vi "Winch Drive.vi"(7 "Description":string, 8 "Command Info In":T1, 10 "Winch Motor":dbl) -> (0 "Command Info Out":T1)   [LabVIEW 2017]
doc: "This template is useful for immediate subsystem actions that do not need deadband filtering\n\nBe sure to right-click and select New from Template and save with a new command name."
uses:
  <vilib>/Rock Robotics/WPI/Framework/Command Status Info.ctl
  <vilib>/Rock Robotics/WPI/Framework/Completion Status.ctl
  <vilib>/Rock Robotics/WPI/Framework/Completion Notifier.ctl
  Implementation/Lift Setpoints.ctl
  Implementation/Lift Operations.ctl
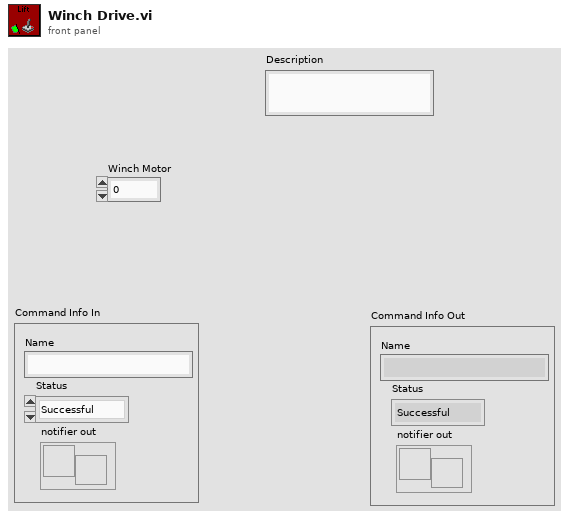
[diagram p1: front panel]
types:
  T1 = typedef "Command Status Info.ctl" = cluster{"Name":string, "Status":T2, "notifier out":T3}
  T2 = typedef "Completion Status.ctl" = enum16{"Successful", "Aborted", "Incomplete"}
  T3 = typedef "Completion Notifier.ctl" = refnum<notifier>
  T4 = typedef "Lift Setpoints.ctl" = cluster{"Operation":T5, "Winch Motor ":dbl, "Hook Motor":dbl}
  T5 = typedef "Lift Operations.ctl" = enum16{"Reserve", "Read Current", "Immediate", "Set Hook Motor", "Set Winch Motor"}
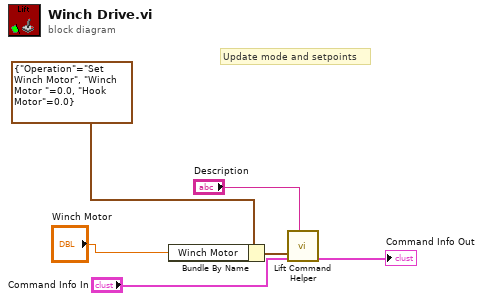
[diagram p0: block diagram]
diagram:
  # "Update mode and setpoints"
  n1 = Bundle By Name(cluster=T4 {"Operation"=enum."Set Winch Motor", "Winch Motor "=0.0, "Hook Motor"=0.0} ("SubSystem Data"), "Winch Motor"="Winch Motor") -> (w2:T4)
  n2 = call "Lift Command Helper.vi"("Description"="Description", "Command Info In"="Command Info In", "SubSystem Data"=w2) -> ("Command Info Out"=→"Command Info Out":T1)  [unwired: 6 in, 2 out]
